vi "ELOG_Calculations_Get.vi"(8 "error in (no error)":errorcluster, 11 "OXY_SCPI Reseource In":refnum<visa-resource-name>) -> (0 "error out":errorcluster, 1 "communication_data":T1, 2 "Calculation Modes":string[](array[string]), 3 "OXY_SCPI Reseource Out":refnum<visa-resource-name>)   [LabVIEW 2018, in "OXYGEN.lvlib"]
doc: "Queries the list of configured calculation modes"
uses:
  OXYGEN.lvlib
  TypeDefs/Cluster_RawCommData.ctl
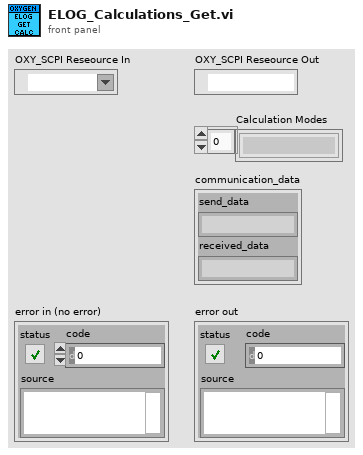
[diagram p1: front panel]
types:
  T1 = typedef "OXYGEN.lvlib/Cluster_RawCommData.ctl" = cluster{"send_data":string, "received_data":string}
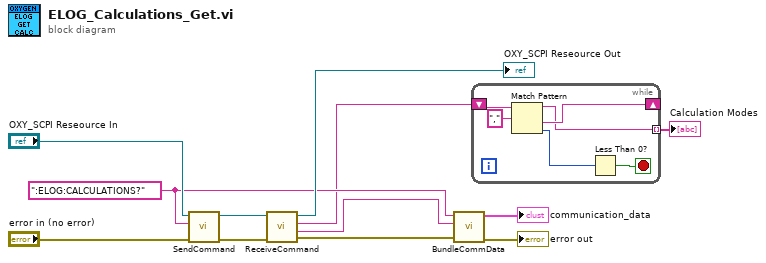
[diagram p0: block diagram]
diagram:
  w4 = ":ELOG:CALCULATIONS?" ("String to Send")
  n1 = call "SendCommand.vi"("error in (no error)"="error in (no error)", "String to Send"=w4, "OXY_SCPI Reseource In"="OXY_SCPI Reseource In") -> ("error out"=w12:errorcluster, "OXY_SCPI Reseource Out"=w11:refnum<visa-resource-name>)  [unwired: 7 in]
  n2 = call "ReceiveCommand.vi"("error in (no error)"=w12, "OXY_SCPI Reseource In"=w11) -> ("error out"=w3:errorcluster, "received Data with Header"=w5:string, "received Data"=w2:string, "OXY_SCPI Reseource Out"=→"OXY_SCPI Reseource Out":refnum<visa-resource-name>)  [unwired: 6 in]
  n3 = call "BundleCommData.vi"("error in (no error)"=w3, "received_data"=w5, "send_data"=w4) -> ("error out"=→"error out":errorcluster, "communication_data"=→"communication_data":T1)  [unwired: 7 in]
  n4 = while {
    shift-right: [w16] -> _
    shift-left: w2 -> [w18]
    tunnel: [w13] -> w1 mode=indexing
    stop <- w14 stop-if-true
    n5 = Match Pattern(string=w18, regular expression=",") -> (before substring=w13:string, after substring=w16:string, offset past match=w15:i32)  [unwired: 1 in, 1 out]
    n6 = Less Than 0?(x=w15) -> (x < 0?=w14:bool)
  }
  "Calculation Modes" <- w1
